vi "Close.vi"(8 "error in (no error)":errorcluster, 11 "State in":T1={"State"=enum."Idle", "Start Time"=timestamp(0 s since 1904-01-01), "Current Time"=timestamp(0 s since 1904-01-01), "First Iteration"=FALSE, "Process Name"="", "Output Error"=FALSE, "Log Started"=FALSE, "Cycle Period"=50.0, "Configuration"={"Valve Settings"={"D-O Settings"={"DAQmx Task Name"="", "Output Channel"=0, "Output Channel Names"=[]}, "VICI Electronic Actuator"={"VISA resource name"="", "Mode"=enum."Two Positions With Stops", "Simulated"=FALSE}}, "Valve Type"=enum."Default", "Time On (Sec)"=0.0, "Time Off (Sec)"=0.0, "Run?"=FALSE}, "Data"={"D-O State"=enum."Off"}} {"Configuration"."Valve Settings"."D-O Settings"."Output Channel" items=["Choose a Channel"]}) -> (0 "error out":errorcluster, 3 "State out":T1={"State"=enum."Idle", "Start Time"=timestamp(0 s since 1904-01-01), "Current Time"=timestamp(0 s since 1904-01-01), "First Iteration"=FALSE, "Process Name"="", "Output Error"=FALSE, "Log Started"=FALSE, "Cycle Period"=50.0, "Configuration"={"Valve Settings"={"D-O Settings"={"DAQmx Task Name"="", "Output Channel"=0, "Output Channel Names"=[]}, "VICI Electronic Actuator"={"VISA resource name"="", "Mode"=enum."Two Positions With Stops", "Simulated"=FALSE}}, "Valve Type"=enum."Default", "Time On (Sec)"=0.0, "Time Off (Sec)"=0.0, "Run?"=FALSE}, "Data"={"D-O State"=enum."Off"}} {"Configuration"."Valve Settings"."D-O Settings"."Output Channel" items=["Choose a Channel"]})   [LabVIEW 2018]
uses:
  State Cluster.ctl
  State Enum.ctl
  Valve Clusters.ctl
  D-O Module Settings Cluster.ctl
  D-O Device Settings Cluster.ctl
  VICI Electronic Actuator/VICI Electronic Actuator Settings.ctl
  D-O Module Engine.lvlib
  D-O Module.lvlib
  DIO Valve/VICI Electronic Actuator.lvlib
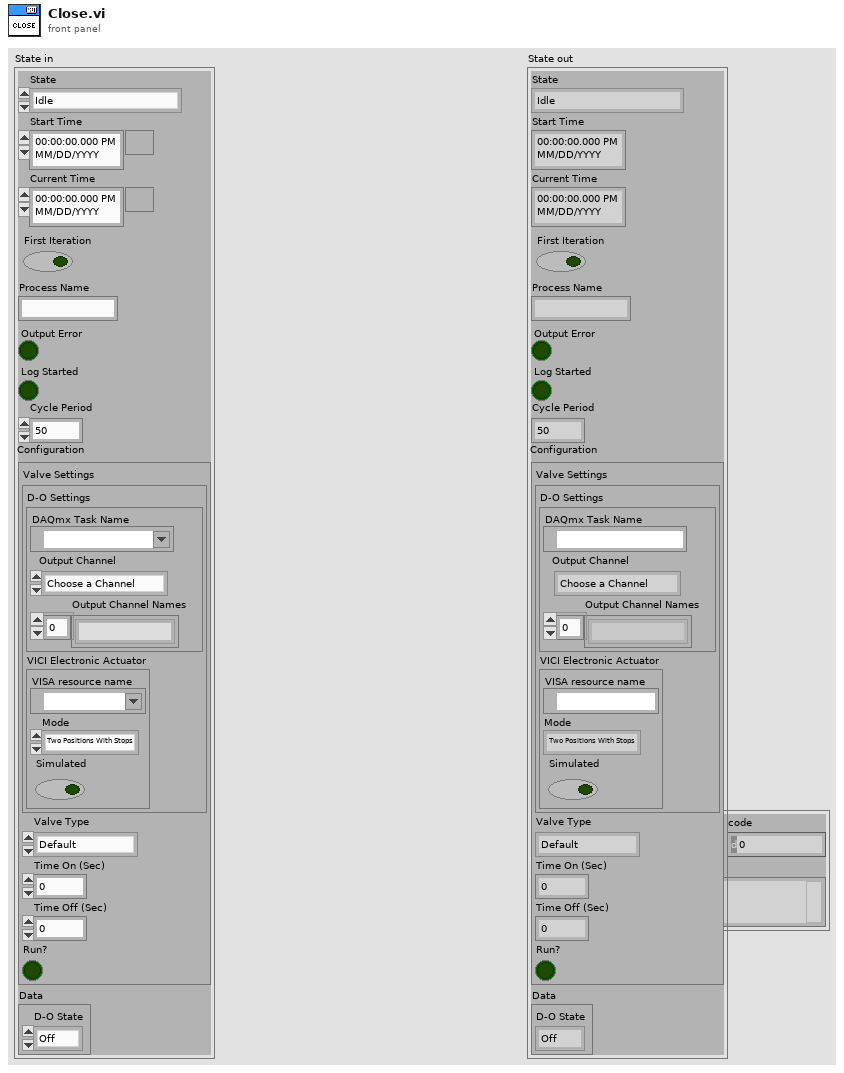
[diagram p1: front panel]
types:
  T1 = typedef "D-O Module.lvlib/D-O Module Engine.lvlib/State Cluster.ctl" = cluster{"State":T2, "Start Time":timestamp, "Current Time":timestamp, "First Iteration":bool, "Process Name":string, "Output Error":bool, "Log Started":bool, "Cycle Period":dbl, "Configuration":T3, "Data":cluster{"D-O State":enum16{"Off", "On", "Not Initialized"}}}
  T2 = typedef "D-O Module.lvlib/D-O Module Engine.lvlib/State Enum.ctl" = enum16{"Measuring", "Idle", "Paused"}
  T3 = typedef "D-O Module.lvlib/Valve Clusters.ctl" = cluster{"Valve Settings":T4, "Valve Type":enum16{"Default", "Digital Output Valve", "VICI Electronic Actuator"}, "Time On (Sec)":dbl, "Time Off (Sec)":dbl, "Run?":bool}
  T4 = typedef "D-O Module.lvlib/D-O Module Settings Cluster.ctl" = cluster{"D-O Settings":T5, "VICI Electronic Actuator":T6}
  T5 = typedef "D-O Module.lvlib/D-O Device Settings Cluster.ctl" = cluster{"DAQmx Task Name":refnum<k21>, "Output Channel":u16, "Output Channel Names":string[]}
  T6 = typedef "VICI Electronic Actuator.lvlib/VICI Electronic Actuator Settings.ctl" = cluster{"VISA resource name":refnum<visa-resource-name>, "Mode":enum16{"Two Positions With Stops", "Two Positions Without Stops", "Mutiposition"}, "Simulated":bool}
  T7 = enum16{"Default", "Digital Output Valve", "VICI Electronic Actuator"}
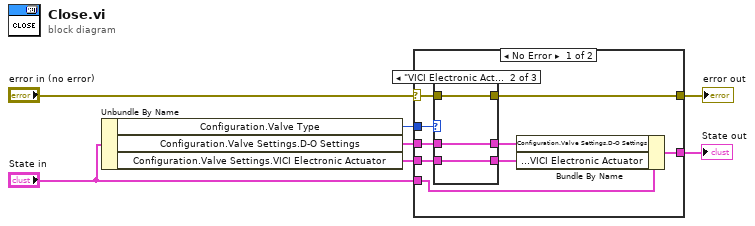
[diagram p0: block diagram]
diagram:
  n1 = Unbundle By Name("State in") -> ("Configuration.Valve Type"=w3:T7, "Configuration.Valve Settings.D-O Settings"=w2:T5, "Configuration.Valve Settings.VICI Electronic Actuator"=w1:T6)
  n2 = case shown="No Error" "error in (no error)" {
    selector: "error in (no error)" -> [w13 w27]
    tunnel: [w14 w27] -> w6
    tunnel: "State in" -> [w16 w26]
    tunnel: [w15 w26] -> w4
    tunnel: w3 -> [w12 _]
    tunnel: w2 -> [w11 _]
    tunnel: w1 -> [w10 _]
    frame No Error {
      n3 = case shown="\"VICI Electronic Actuator\"" w12 {
        tunnel: w11 -> [w17 w21 w25]
        tunnel: [w17 w21 w25] -> w9
        tunnel: w10 -> [w18 w22 w23]
        tunnel: [w19 w20 w24] -> w14
        tunnel: w13 -> [w19 w20 w24]
        tunnel: [w18 w22 w23] -> w8
        frame "Digital Output Valve" {
        }
        frame "VICI Electronic Actuator" {
        }
        frame "Default", Default {
        }
      }
      n4 = Bundle By Name(cluster=w16, "Configuration.Valve Settings.D-O Settings"=w9, "Configuration.Valve Settings.VICI Electronic Actuator"=w8) -> (w15:T1)
    }
    frame Error {
    }
  }
  "error out" <- w6
  "State out" <- w4
